vi "Write Exit.vi"(8 "error in (no error)":errorcluster, 10 "Exit":bool, 11 "AbstractionMessage in":refnum<class "AbstractionMessage.lvclass">) -> (0 "error out":errorcluster, 3 "AbstractionMessage out":refnum<class "AbstractionMessage.lvclass">)   [LabVIEW 2014, in "AbstractionMessage.lvclass"]
uses:
  AbstractionMessage.lvclass
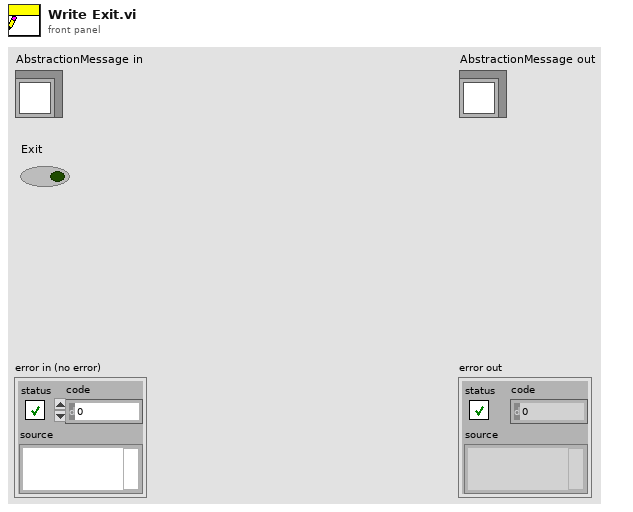
[diagram p1: front panel]
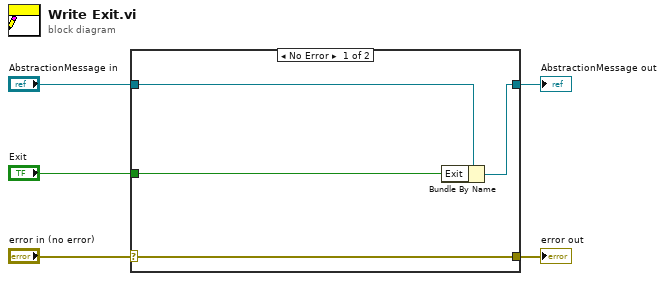
[diagram p0: block diagram]
diagram:
  n1 = case shown="No Error" "error in (no error)" {
    selector: "error in (no error)" -> [w9 w10]
    tunnel: [w9 w10] -> w4
    tunnel: [w7 w11] -> w2
    tunnel: "AbstractionMessage in" -> [w8 w11]
    tunnel: "Exit" -> [w6 _]
    frame No Error {
      n2 = Bundle By Name(cluster=w8, "Exit"=w6) -> (w7:refnum<class "AbstractionMessage.lvclass">)
    }
    frame Error {
    }
  }
  "error out" <- w4
  "AbstractionMessage out" <- w2
